vi "Read RD Data Queue.vi"(8 "error in (no error)":errorcluster, 11 "tCRD in":refnum<class "tCRD.lvclass">) -> (0 "error out":errorcluster, 2 "RD Data Queue":refnum<queue>, 3 "tCRD out":refnum<class "tCRD.lvclass">)   [LabVIEW 2013]
uses:
  tCRD.lvclass
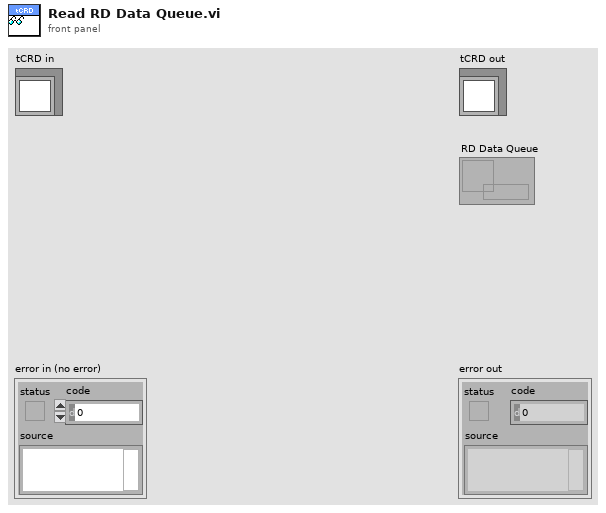
[diagram p1: front panel]
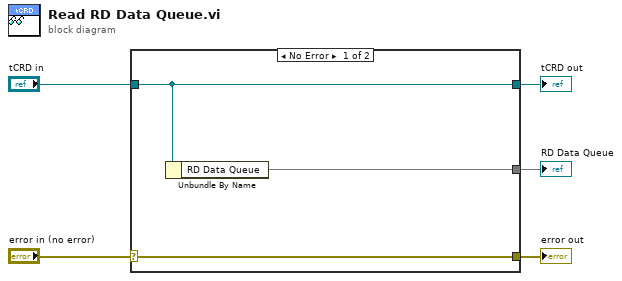
[diagram p0: block diagram]
diagram:
  n1 = case shown="No Error" "error in (no error)" {
    selector: "error in (no error)" -> [w8 w9]
    tunnel: [w8 w9] -> w4
    tunnel: [w7 w10] -> w2
    tunnel: "tCRD in" -> [w7 w10]
    tunnel: [w6 _] -> w1
    frame No Error {
      n2 = Unbundle By Name(w7) -> ("RD Data Queue"=w6)
    }
    frame Error {
    }
  }
  "error out" <- w4
  "tCRD out" <- w2
  "RD Data Queue" <- w1
